vi "vi.VariantToClusterArray.vi"(0 "ClusterArray":variant, 11 "error in":errorcluster) -> (4 "VariantArray":variant[](array[variant]), 15 "error out":errorcluster)   [LabVIEW 2014, in "GLue.lvlib" / "class.GLue.lvclass"]
uses:
  class.GLue.lvclass
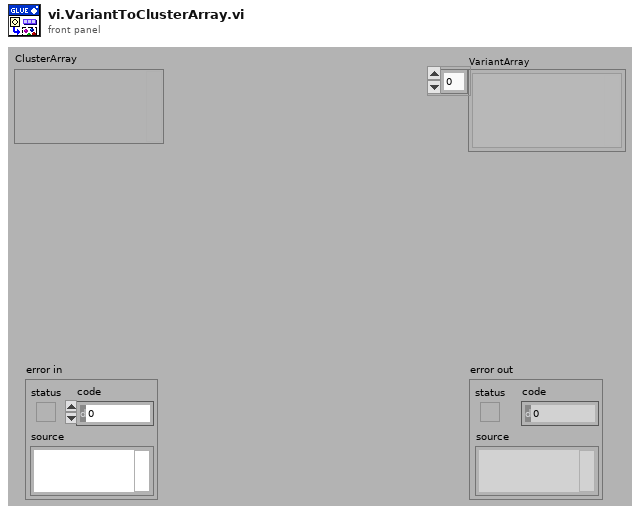
[diagram p1: front panel]
types:
  T1 = enum8{"<Null>", "I8", "I16", "I32", "I64", "U8", "U16", "U32", "U64", "SGL", "DBL", "EXT", "CSG", "CDB", "CXT", "0x0F", "0x10", "0x11", "0x12", "0x13", "0x14", "Enum U8", "Enum U16", "Enum U32", "Enum U64", "SGL PQ", "DBL PQ", "EXT PQ", "CSG PQ", "CDB PQ", "CXT PQ", "0x1F", "0x20", "Boolean", "0x22", "0x23", "0x24", "0x25", "0x26", "0x27", "0x28", "0x29", "0x2A", "0x2B", "0x2C", "0x2D", "0x2E", "0x2F", "String", "0x31", "Path", "Pict", "0x34", "0x35", "0x36", "DAQ", "0x38", "0x39", "0x3A", "0x3B", "0x3C", "0x3D", "0x3E", "0x3F", "Array", "0x41", "0x42", "0x43", "0x44", "0x45", "0x46", "0x47", "0x48", "0x49", "0x4A", "0x4B", "0x4C", "0x4D", "0x4E", "0x4F", "Cluster", "0x51", "0x52", "Variant", "Waveform", "0x55", "0x56", "0x57", "0x58", "0x59", "0x5A", "0x5B", "0x5C", "0x5D", "0x5E", "0x5F", "0x60", "0x61", "0x62", "0x63", "0x64", "0x65", "0x66", "0x67", "0x68", "0x69", "0x6A", "0x6B", "0x6C", "0x6D", "0x6E", "0x6F", "Refnum"}
  T2 = cluster{"length":u16, "private":u8, "type":enum8{"<Null>", "I8", "I16", "I32", "I64", "U8", "U16", "U32", "U64", "SGL", "DBL", "EXT", "CSG", "CDB", "CXT", "0x0F", "0x10", "0x11", "0x12", "0x13", "0x14", "Enum U8", "Enum U16", "Enum U32", "Enum U64", "SGL PQ", "DBL PQ", "EXT PQ", "CSG PQ", "CDB PQ", "CXT PQ", "0x1F", "0x20", "Boolean", "0x22", "0x23", "0x24", "0x25", "0x26", "0x27", "0x28", "0x29", "0x2A", "0x2B", "0x2C", "0x2D", "0x2E", "0x2F", "String", "0x31", "Path", "Pict", "0x34", "0x35", "0x36", "DAQ", "0x38", "0x39", "0x3A", "0x3B", "0x3C", "0x3D", "0x3E", "0x3F", "Array", "0x41", "0x42", "0x43", "0x44", "0x45", "0x46", "0x47", "0x48", "0x49", "0x4A", "0x4B", "0x4C", "0x4D", "0x4E", "0x4F", "Cluster", "0x51", "0x52", "Variant", "Waveform", "0x55", "0x56", "0x57", "0x58", "0x59", "0x5A", "0x5B", "0x5C", "0x5D", "0x5E", "0x5F", "0x60", "0x61", "0x62", "0x63", "0x64", "0x65", "0x66", "0x67", "0x68", "0x69", "0x6A", "0x6B", "0x6C", "0x6D", "0x6E", "0x6F", "Refnum"}, "# elements":u16}
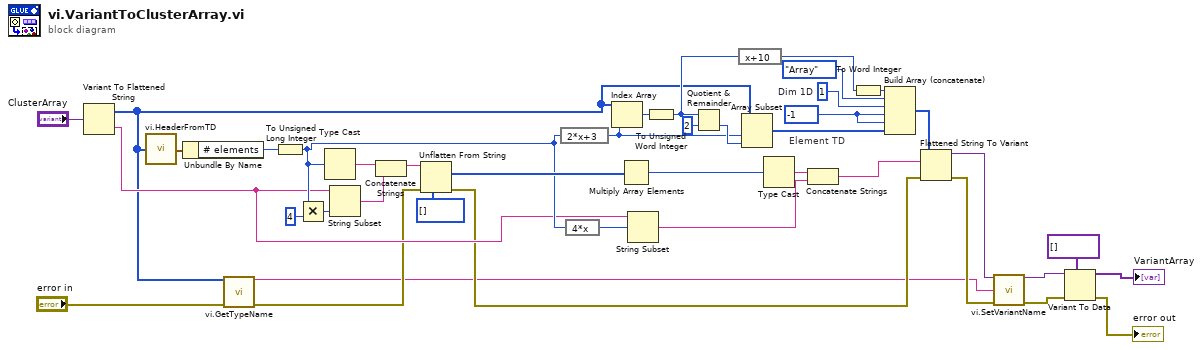
[diagram p0: block diagram]
diagram:
  w23 = i16 -1 ("Input Element")
  w19 = i16 1  # Dim 1D
  # "Element TD"
  n1 = Variant To Flattened String(Variant="ClusterArray") -> (data string=w13:string, 1:w10:i16[])
  n2 = call "vi.HeaderFromTD.vi"("Type Descriptor"=w10) -> ("Type Descriptor Header"=w34:T2)  [unwired: 4 in]
  n3 = Unbundle By Name(w34) -> ("# elements"=w33:u16)
  n4 = call "vi.GetTypeName.vi"("Type Descriptor"=w10, "error in"="error in") -> ("Name"=w6:string, "error out"=w11:errorcluster)  [unwired: 12 in]
  n5 = To Unsigned Long Integer(number=w33) -> (unsigned 32bit integer=w14:u32)
  n6 = Multiply(x=w14, y=u32 4) -> (x*y=w37:u32)
  n7 = Type Cast(x=w14) -> (*(type *) &x=w40:string)  [unwired: 1 in]
  n8 = String Subset(string=w13, length (rest)=w37) -> (substring=w39:string)  [unwired: 1 in]
  n9 = Concatenate Strings(w40, w39) -> (w38:string)
  n10 = Unflatten From String(type=u32[] [] ("Size(s)"), binary string=w38, error in (no error)=w11) -> (value=w15:u32[], error out=w9:errorcluster)  [unwired: 2 in, 1 out]
  n11 = expression code="2*x+3"(w14) -> (w16:u32)
  n12 = expression code="4*x"(w14) -> (w24:u32)
  n13 = Index Array(array=w10, index=w16) -> (element=w22:i16)
  n14 = Multiply Array Elements(1:w15) -> (0:w25:u32)
  n15 = String Subset(string=w13, offset (0)=w24) -> (substring=w27:string)  [unwired: 1 in]
  n16 = To Unsigned Word Integer(number=w22) -> (unsigned 16bit integer=w30:u16)
  n17 = Quotient & Remainder(x=w30, y=u16 2) -> (floor(x/y)=w21:u16)  [unwired: 1 out]
  n18 = expression code="x+10"(w30) -> (w20:u16)
  n19 = Array Subset(array=w10, index=w16, length=w21) -> (w18:i16[])
  n20 = Type Cast(x=w25) -> (*(type *) &x=w26:string)  [unwired: 1 in]
  n21 = Concatenate Strings(w26, w27) -> (w29:string)
  n22 = To Word Integer(number=w20) -> (16bit integer=w31:i16)
  n23 = Build Array (concatenate)(w31, T1."Array" ("Type Descriptor Enumeration"), w19, w23, w23, w18) -> (w28:i16[])
  n24 = Flattened String To Variant(4:w9, 6:w29, 7:w28) -> (0:w8:errorcluster, 3:w7:variant)
  n25 = call "vi.SetVariantName.vi"("Variant in"=w7, "Name"=w6, "error in"=w8) -> ("Named Variant"=w4:variant, "error out"=w3:errorcluster)  [unwired: 11 in]
  n26 = Variant To Data(error in=w3, type=variant[] [], Variant=w4) -> (data=→"VariantArray":variant[], error out=→"error out":errorcluster)
